vi "Temperature Controller.vi"(8 "Launch Order":i32, 9 "My Name":string) -> ()   [LabVIEW 2020, in "Startup Processes.lvlib"]
uses:
  Startup Processes.lvlib
  _typedefs/State Machine Conditions.ctl
  _typedefs/Machine Modes.ctl
  _typedefs/Subpanel Names.ctl
  _typedefs/States.ctl
  _ude/Change Source/_subVIs/Get Event Reference.vi
  toolbox/Standard Signalling/ude_Stop Application/Get Event Reference.vi
  toolbox/Standard Signalling/ude_Stop Application/ude_Stop Application.lvlib
  toolbox/Standard Signalling/ude_Handle Errors/ude_Handle Errors.lvlib
  _ude/Change Source/Change Source.lvlib
  _buffers/Plugin References/Plugin References.lvlib
  toolbox/User Interface/User Interface.lvlib
  Display Properties Manager/Display Properties Manager.lvlib
  _buffers/Temperature Controller Data Buffer/Temperature Controller Data Buffer.lvlib
  _buffers/Plugin Chart References/Plugin Chart References.lvlib
  _ude/Read Graph Data/Read Graph Data.lvlib
panel:
  out "Cooler":bool
  out "Fan":bool
  out "Data":T1(graph)
  out "Error Out":errorcluster
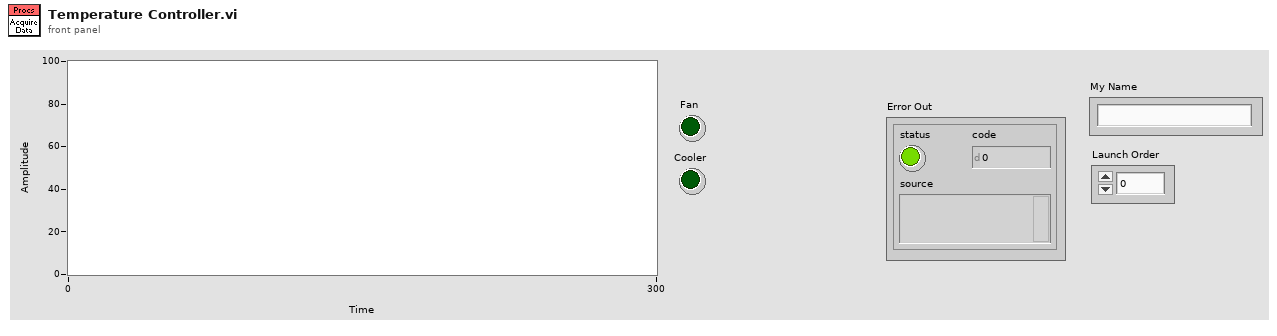
[diagram p1: front panel]
types:
  T1 = cluster{"Last value":dbl, "Error High Level":dbl, "Warning High Level":dbl, "Warning Low Level":dbl, "Error Low Level":dbl}
  T2 = typedef "Startup Processes.lvlib/Subpanel Names.ctl" = enum16{"Sine Source", "Ramp Source", "Hen House TC", "Dog House TC", "Out House TC"}
  T3 = typedef "Startup Processes.lvlib/State Machine Conditions.ctl" = cluster{"Last value":dbl, "Last Sample Time":dbl[unit], "Fan State":enum16{"Off", "On"}, "Cooler State":enum16{"Off", "On"}, "Timeout":i32, "Mode":T4, "Machine Name":T2}
  T4 = typedef "Startup Processes.lvlib/Machine Modes.ctl" = enum16{"Startup", "Run"}
  T5 = cluster{"reuse":refnum<event-registration>, "daq":refnum<event-registration>, "sys":refnum<event-registration>}
  T6 = typedef "Startup Processes.lvlib/States.ctl" = enum16{"Initialization", "Read Input", "Test Fan Limits", "Set Fan", "Test Cooler Limits", "Set Cooler", "Acquisition TO Wait", "Error", "Deinitialize"}
  T7 = cluster{"Last value":dbl, "Error High Level":dbl, "Warning High Level":dbl, "Warning Low Level":dbl, "Error Low Level":dbl}[]
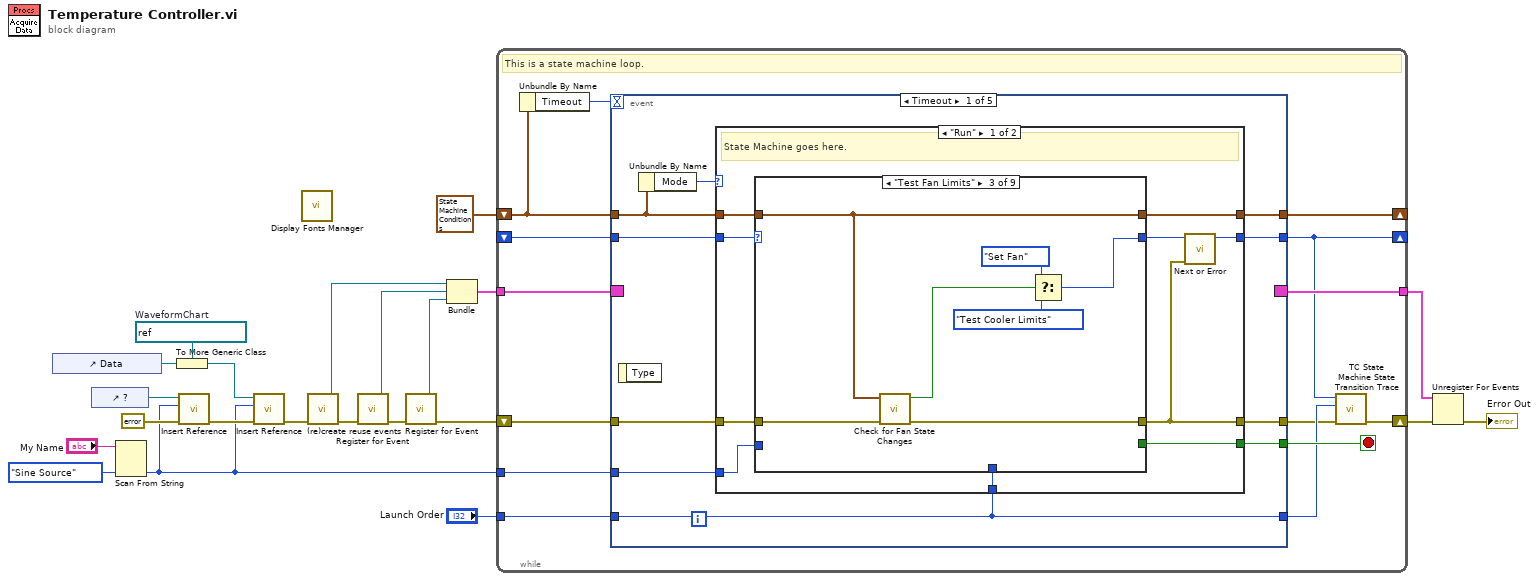
[diagram p0: block diagram]
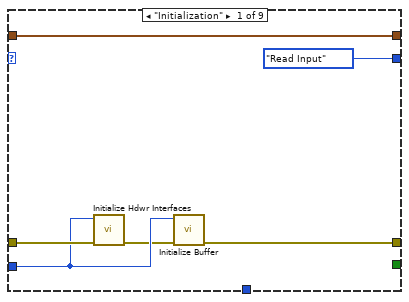
[diagram p2: hidden frame]
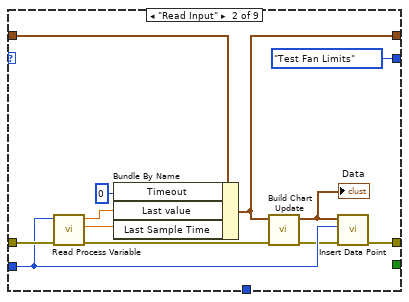
[diagram p3: hidden frame]
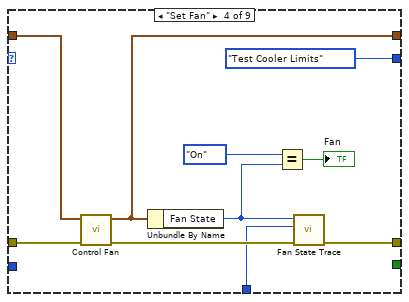
[diagram p4: hidden frame]
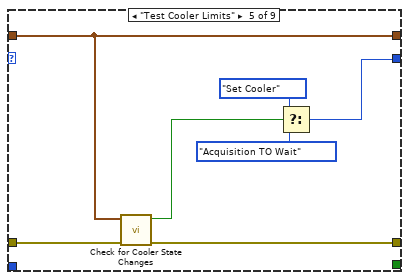
[diagram p5: hidden frame]
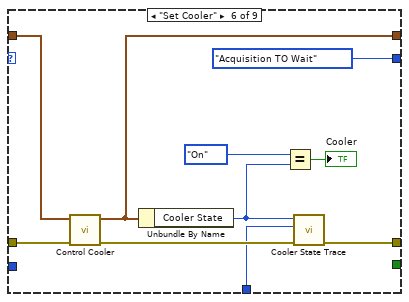
[diagram p6: hidden frame]
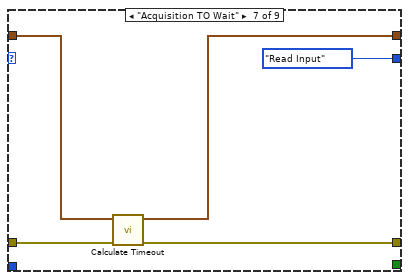
[diagram p7: hidden frame]
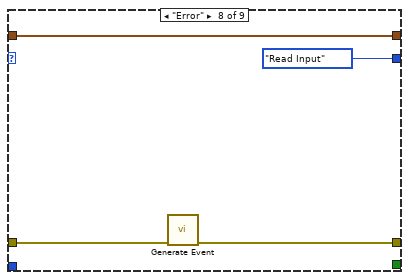
[diagram p8: hidden frame]
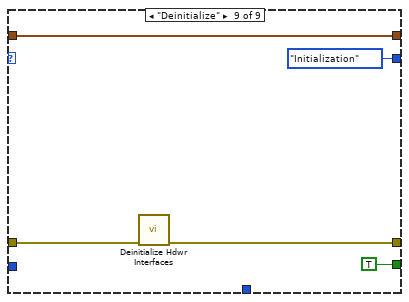
[diagram p9: hidden frame]
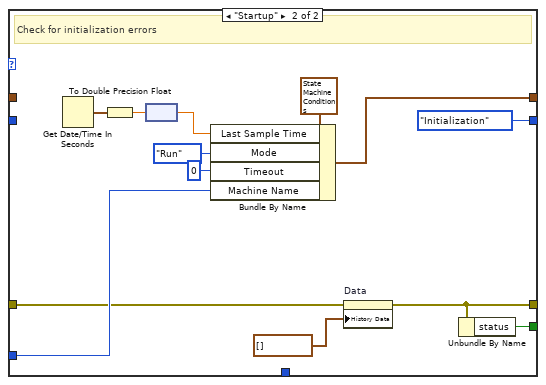
[diagram p10: hidden frame]
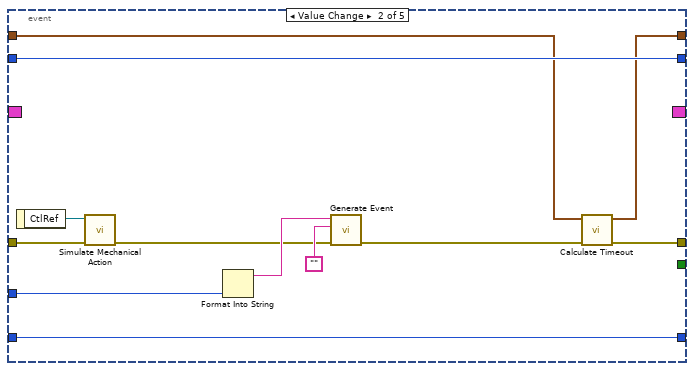
[diagram p11: hidden frame]
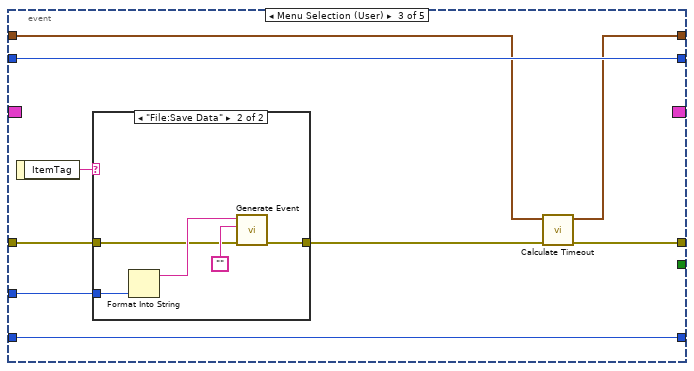
[diagram p12: hidden frame]
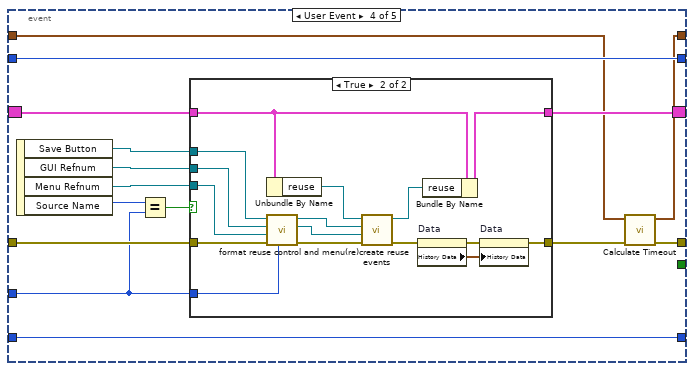
[diagram p14: hidden frame]
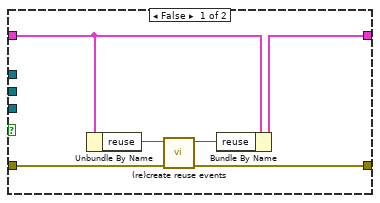
[diagram p15: hidden frame]
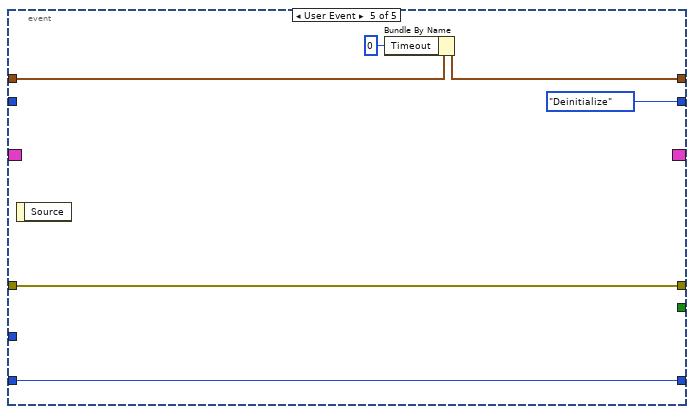
[diagram p16: hidden frame]
diagram:
  w7 = refnum<vi> refnum  # WaveformChart
  n1 = control-ref of="Data"() -> (w4:refnum<vi>)
  n2 = control-ref of="?"() -> (w14:refnum<vi>)
  n3 = Scan From String(input string="My Name", default 1=Subpanel_Names."Sine Source" ("Plugin Names")) -> (output 1=w1:T2)  [unwired: 3 in, 3 out]
  n4 = To More Generic Class(target class=w7, reference=w4) -> (generic class reference=w8:refnum<vi>)
  n5 = call "Insert Reference.vi"("Error In"=errorcluster {"status"=FALSE, "code"=0, "source"=""} ("Error Out"), "Plugin Name"=w1, "VI Refnum"=w14) -> ("Error Out"=w6:errorcluster)  [unwired: 4 in]
  n6 = call "Insert Reference.vi"("Error In"=w6, "Plugin Name"=w1, "WFChart Refnum"=w8) -> ("Error Out"=w5:errorcluster)  [unwired: 4 in]
  n7 = call "Display Fonts Manager.vi"() -> ()  [unwired: 7 in, 1 out]
  n8 = call "(re)create reuse events.vi"("error in (no error)"=w5) -> ("error out"=w12:errorcluster, "reuse"=w11:refnum<event-registration>)  [unwired: 5 in]
  n9 = call "Register for Event.vi"("Error In"=w12) -> ("Error Out"=w15:errorcluster, "daq"=w16:refnum<event-registration>)  [unwired: 5 in]
  n10 = call "Register for Event.vi"("Error In"=w15) -> ("Error Out"=w19:errorcluster, "sys"=w21:refnum<event-registration>)  [unwired: 5 in]
  n11 = Bundle("reuse"=w11, "daq"=w16, "sys"=w21) -> (w17:T5)  [unwired: 1 in]
  n12 = while {
    shift-right: [w23] -> w22
    shift-left: w19 -> [w36]
    tunnel: w17 -> [w35]
    tunnel: [w34] -> w20
    shift-right: [w31] -> _
    shift-left: T3 {"Last value"=0.0, "Last Sample Time"=0.0, "Fan State"=enum."Off", "Cooler State"=enum."Off", "Timeout"=0, "Mode"=enum."Startup", "Machine Name"=enum."Sine Source"} ("State Machine Data") -> [w32]
    tunnel: w1 -> [w30]
    shift-right: [w24] -> _
    shift-left: _ -> [w29]
    tunnel: "Launch Order" -> [w27]
    stop <- w33 stop-if-true
    # "This is a state machine loop."
    n13 = Unbundle By Name(w32) -> ("Timeout"=w28:i32)
    n14 = event shown="[0] Timeout" {
      selector: w35 -> [_ _ _ w171 _]
      dyn-events: [_ _ _ w170 _] -> w34
      timeout: w28 -> [_ _ _ _ _]
      tunnel: w36 -> [w46 w147 w155 w176 w205]
      tunnel: [w38 w142 w149 w167 w205] -> w25
      tunnel: [w44 _ _ _ _] -> w33
      tunnel: w32 -> [w41 w144 w152 w169 w203]
      tunnel: [w45 w143 w151 w168 w202] -> w31
      tunnel: w30 -> [w40 w137 w154 w164 _]
      tunnel: w29 -> [w43 w145 w153 w172 _]
      tunnel: [w39 w145 w153 w172 States."Deinitialize" ("States")] -> w24
      tunnel: w27 -> [w37 w141 w148 w165 w200]
      tunnel: [w37 w141 w148 w165 w200] -> w26
      event Timeout {
        n15 = event-data() -> ()  [unwired: 1 in, 1 out]
        n16 = Unbundle By Name(w41) -> ("Mode"=w42:T4)
        n17 = case shown="\"Run\"" w42 {
          tunnel: [w50 w132] -> w38
          tunnel: [w56 w125] -> w45
          tunnel: [w49 w135] -> w44
          tunnel: w46 -> [w53 w123]
          tunnel: w41 -> [w55 _]
          tunnel: w43 -> [w54 _]
          tunnel: [w51 States."Initialization" ("States")] -> w39
          tunnel: w40 -> [w48 w124]
          tunnel: w37 -> [w47 _]
          frame "Run" {
            # "State Machine goes here."
            n18 = case shown="\"Test Fan Limits\"" w54 {
              tunnel: [w62 w68 w79 w88 w96 w105 w109 w117 w122] -> w56
              tunnel: w55 -> [w62 w69 w79 w91 w96 w108 w110 w117 w122]
              tunnel: [w57 w67 w80 w84 w97 w101 w111 w114 w118] -> w50
              tunnel: w53 -> [w61 w74 w81 w90 w98 w107 w112 w115 w119]
              tunnel: [States."Read Input" ("States") States."Test Fan Limits" ("States") w77 States."Test Cooler Limits" ("States") w92 States."Acquisition TO Wait" ("States") States."Read Input" ("States") States."Read Input" ("States") States."Initialization" ("States")] -> w52
              tunnel: [_ _ _ _ _ _ _ _ TRUE] -> w49
              tunnel: w48 -> [w59 w65 _ _ _ _ _ _ _]
              tunnel: w47 -> [_ _ _ w82 _ w99 _ _ _]
              frame "Initialization" {
                n19 = call "Initialize Hdwr Interfaces.vi"("error in (no error)"=w61, "Instance Name"=w59) -> ("error out"=w58:errorcluster)  [unwired: 5 in]
                n20 = call "Initialize Buffer.vi"("Error In"=w58, "Instance Name"=w59) -> ("Error Out"=w57:errorcluster)  [unwired: 5 in]
              }
              frame "Read Input" {
                n21 = call "Read Process Variable.vi"("error in (no error)"=w74, "Instance Name"=w65) -> ("error out"=w64:errorcluster, "Last Sample Time"=w70:dbl[unit], "Last value"=w73:dbl)  [unwired: 3 in]
                n22 = Bundle By Name(cluster=w69, "Timeout"=0, "Last value"=w73, "Last Sample Time"=w70) -> (w68:T3)
                n23 = call "Build Chart Update.vi"("error in (no error)"=w64, "State Machine Data"=w68) -> ("error out"=w63:errorcluster, "Chart Sample"=w66:T1)  [unwired: 4 in]
                "Data" <- w66
                n24 = call "Insert Data Point.vi"("Error In"=w63, "Instance Name"=w65, "Data"=w66) -> ("Error Out"=w67:errorcluster)  [unwired: 4 in]
              }
              frame "Test Fan Limits" {
                n25 = call "Check for Fan State Changes.vi"("error in (no error)"=w81, "State Machine Data"=w79) -> ("error out"=w80:errorcluster, "Toggle Fan State?"=w75:bool)  [unwired: 4 in]
                n26 = Select(t=States."Set Fan" ("States"), s=w75, f=States."Test Cooler Limits" ("States")) -> (s? t:f=w77:T6)
              }
              frame "Set Fan" {
                n27 = call "Control Fan.vi"("error in (no error)"=w90, "State Machine Data in"=w91) -> ("error out"=w85:errorcluster, "State Machine Data out"=w88:T3)  [unwired: 4 in]
                n28 = Unbundle By Name(w88) -> ("Fan State"=w83:enum16{"Off", "On"})
                n29 = Equal?(x=enum16{"Off", "On"}."On" ("y"), y=w83) -> (x = y?=→"Fan":bool)
                n30 = call "Fan State Trace.vi"("error in (no error)"=w85, "Launch Order"=w82, "Fan State"=w83) -> ("error out"=w84:errorcluster)  [unwired: 4 in]
              }
              frame "Test Cooler Limits" {
                n31 = call "Check for Cooler State Changes.vi"("error in (no error)"=w98, "State Machine Data"=w96) -> ("error out"=w97:errorcluster, "Cooler Need Adjusting?"=w93:bool)  [unwired: 4 in]
                n32 = Select(t=States."Set Cooler" ("States"), s=w93, f=States."Acquisition TO Wait" ("States")) -> (s? t:f=w92:T6)
              }
              frame "Set Cooler" {
                n33 = call "Control Cooler.vi"("error in (no error)"=w107, "State Machine Data in"=w108) -> ("error out"=w102:errorcluster, "State Machine Data out"=w105:T3)  [unwired: 4 in]
                n34 = Unbundle By Name(w105) -> ("Cooler State"=w100:enum16{"Off", "On"})
                n35 = Equal?(x=enum16{"Off", "On"}."On" ("y"), y=w100) -> (x = y?=→"Cooler":bool)
                n36 = call "Cooler State Trace.vi"("error in (no error)"=w102, "Launch Order"=w99, "Cooler State"=w100) -> ("error out"=w101:errorcluster)  [unwired: 4 in]
              }
              frame "Acquisition TO Wait" {
                n37 = call "Calculate Timeout.vi"("error in (no error)"=w112, "State Machine Data in"=w110) -> ("error out"=w111:errorcluster, "State Machine Data out"=w109:T3)  [unwired: 4 in]
              }
              frame "Error" {
                n38 = call "Generate Event.vi"("Error In"=w115) -> ("Error Out"=w114:errorcluster)  [unwired: 6 in]
              }
              frame "Deinitialize" {
                n39 = call "Deinitialize Hdwr Interfaces.vi"("error in (no error)"=w119) -> ("error out"=w118:errorcluster)  [unwired: 6 in]
              }
            }
            n40 = call "Next or Error.vi"("error in (no error)"=w50, "State in"=w52) -> ("State out"=w51:T6)  [unwired: 5 in]
          }
          frame "Startup" {
            # "Check for initialization errors"
            n41 = Get Date/Time In Seconds() -> (seconds since 1Jan1904=w128:timestamp)
            n42 = To Double Precision Float(number=w128) -> (double precision float=w127:dbl)
            n43 = node(w127) -> (w126:dbl[unit])
            n44 = Bundle By Name(cluster=T3 {"Last value"=0.0, "Last Sample Time"=0.0, "Fan State"=enum."Off", "Cooler State"=enum."Off", "Timeout"=0, "Mode"=enum."Startup", "Machine Name"=enum."Sine Source"} ("State Machine Data"), "Last Sample Time"=w126, "Mode"=Machine_Modes."Run", "Timeout"=0, "Machine Name"=w124) -> (w125:T3)
            n45 = property on="Data" class="WFChart (strict)"(error in=w123, "History Data"=T7 []) -> (error out=w132:errorcluster)  [unwired: 1 in, 1 out]
            n46 = Unbundle By Name(w132) -> ("status"=w135:bool)
          }
        }
      }
      event Value Change {
        n47 = event-data() -> ("CtlRef"=w146:refnum<vi>)  [unwired: 1 in]
        n48 = call "Simulate Mechanical Action.vi"("Error In"=w147, "Button CtlRef"=w146) -> ("Error Out"=w138:errorcluster)  [unwired: 5 in]
        n49 = Format Into String(w137) -> (resulting string=w140:string)  [unwired: 3 in, 1 out]
        n50 = call "Generate Event.vi"("Error In"=w138, "Response Notifier"="", "Graph Name"=w140) -> ("Error Out"=w136:errorcluster)  [unwired: 4 in]
        n51 = call "Calculate Timeout.vi"("error in (no error)"=w136, "State Machine Data in"=w144) -> ("error out"=w142:errorcluster, "State Machine Data out"=w143:T3)  [unwired: 4 in]
      }
      event Menu Selection (User) {
        n52 = event-data() -> ("ItemTag"=w156:string)  [unwired: 1 in]
        n53 = case shown="\"File:Save Data\"" w156 {
          tunnel: w155 -> [w157 w160]
          tunnel: [w157 w158] -> w150
          tunnel: w154 -> [_ w159]
          frame Default {
          }
          frame "File:Save Data" {
            n54 = Format Into String(w159) -> (resulting string=w162:string)  [unwired: 3 in, 1 out]
            n55 = call "Generate Event.vi"("Error In"=w160, "Response Notifier"="", "Graph Name"=w162) -> ("Error Out"=w158:errorcluster)  [unwired: 4 in]
          }
        }
        n56 = call "Calculate Timeout.vi"("error in (no error)"=w150, "State Machine Data in"=w152) -> ("error out"=w149:errorcluster, "State Machine Data out"=w151:T3)  [unwired: 4 in]
      }
      event User Event {
        n57 = event-data() -> ("Save Button"=w175:refnum<vi>, "GUI Refnum"=w174:refnum<vi>, "Menu Refnum"=w173:refnum<k9>, "Source Name"=w163:T2)  [unwired: 1 in]
        n58 = Equal?(x=w163, y=w164) -> (x = y?=w177:bool)
        n59 = case shown="True" w177 {
          tunnel: [w179 w189] -> w170
          tunnel: w176 -> [w183 w199]
          tunnel: [w182 w184] -> w166
          tunnel: w175 -> [_ w197]
          tunnel: w174 -> [_ w195]
          tunnel: w173 -> [_ w198]
          tunnel: w164 -> [_ w193]
          tunnel: w171 -> [w180 w190]
          frame False {
            n60 = Unbundle By Name(w180) -> ("reuse"=w181:refnum<event-registration>)
            n61 = call "(re)create reuse events.vi"("error in (no error)"=w183, "reuse in"=w181) -> ("error out"=w182:errorcluster, "reuse"=w178:refnum<event-registration>)  [unwired: 4 in]
            n62 = Bundle By Name(cluster=w180, "reuse"=w178) -> (w179:T5)
          }
          frame True {
            n63 = Unbundle By Name(w190) -> ("reuse"=w192:refnum<event-registration>)
            n64 = call "format reuse control and menu.vi"("My Name"=w193, "error in (no error)"=w199, "Menu Refnum"=w198, "GUI Refnum in"=w195, "Save Button"=w197) -> ("error out"=w186:errorcluster, "GUI Refnum out"=w194:refnum<vi>, "Save Button Out"=w196:refnum<vi>)  [unwired: 1 in]
            n65 = call "(re)create reuse events.vi"("error in (no error)"=w186, "Save Menu"=w194, "Save Button"=w196, "reuse in"=w192) -> ("error out"=w185:errorcluster, "reuse"=w191:refnum<event-registration>)  [unwired: 2 in]
            n66 = property on="Data" class="WFChart (strict)"(error in=w185) -> (error out=w187:errorcluster, "History Data"=w188:T7)  [unwired: 1 in, 1 out]
            n67 = Bundle By Name(cluster=w190, "reuse"=w191) -> (w189:T5)
            n68 = property on="Data" class="WFChart (strict)"(error in=w187, "History Data"=w188) -> (error out=w184:errorcluster)  [unwired: 1 in, 1 out]
          }
        }
        n69 = call "Calculate Timeout.vi"("error in (no error)"=w166, "State Machine Data in"=w169) -> ("error out"=w167:errorcluster, "State Machine Data out"=w168:T3)  [unwired: 4 in]
      }
      event User Event {
        n70 = event-data() -> ()  [unwired: 1 in, 1 out]
        n71 = Bundle By Name(cluster=w203, "Timeout"=0) -> (w202:T3)
      }
    }
    n72 = call "TC State Machine State Transition Trace.vi"("error in (no error)"=w25, "Launch Order"=w26, "Next State"=w24) -> ("error out"=w23:errorcluster)  [unwired: 4 in]
  }
  n73 = Unregister For Events(event registration refnum=w20, error in=w22) -> (error out=→"Error Out":errorcluster)
